vi "Generate_Voice_Event.vi"(8 "Error In":errorcluster, 11 "String in":refnum<vi>) -> (0 "Error Out":errorcluster, 3 "String out":refnum<vi>)   [LabVIEW 2018]
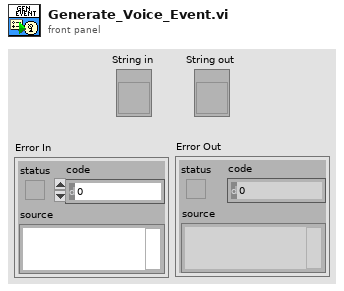
[diagram p1: front panel]
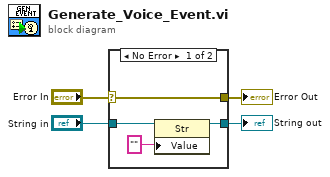
[diagram p0: block diagram]
diagram:
  n1 = case shown="No Error" "Error In" {
    selector: "Error In" -> [w5 w10]
    tunnel: "String in" -> [w8 w9]
    tunnel: [w7 w9] -> w3
    tunnel: [w5 w10] -> w1
    frame No Error {
      n2 = property class="Str"(reference=w8, "Value"="") -> (reference out=w7:refnum<vi>)  [unwired: 1 in, 1 out]
    }
    frame Error {
    }
  }
  "String out" <- w3
  "Error Out" <- w1
